vi "Read GUIs.vi"(8 "error in (no error)":errorcluster, 11 "GUI Composition in":refnum<class "GUI Composition.lvclass">) -> (0 "error out":errorcluster, 2 "GUIs":refnum<class "GUI.lvclass">[](array[class]), 3 "GUI Composition out":refnum<class "GUI Composition.lvclass">)   [LabVIEW 2018, in "GUI Composition.lvclass"]
uses:
  GUI Composition.lvclass
  GUI.lvclass
  GUI Composition.lvclass/GUI Composition.ctl
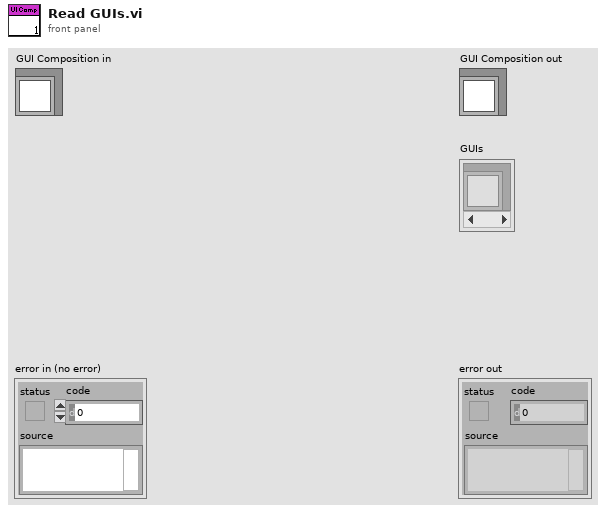
[diagram p1: front panel]
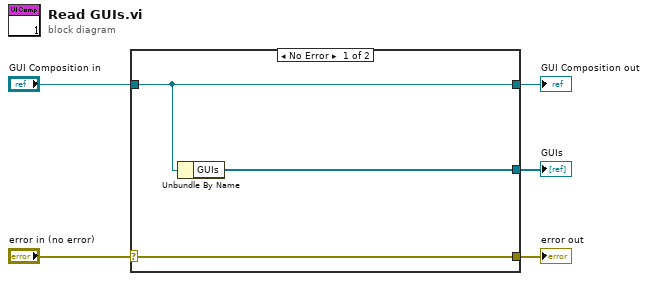
[diagram p0: block diagram]
diagram:
  n1 = case shown="No Error" "error in (no error)" {
    selector: "error in (no error)" -> [w8 w9]
    tunnel: [w8 w9] -> w4
    tunnel: [w7 w10] -> w2
    tunnel: "GUI Composition in" -> [w7 w10]
    tunnel: [w6 _] -> w1
    frame No Error {
      n2 = Unbundle By Name(w7) -> ("GUIs"=w6:refnum<class "GUI.lvclass">[])
    }
    frame Error {
    }
  }
  "error out" <- w4
  "GUI Composition out" <- w2
  "GUIs" <- w1
